vi "Get Transceivers Directory.vi"(8 "error in (no error)":errorcluster, 11 "Transceiver Loader in":refnum<class "Transceiver Loader.lvclass">) -> (0 "error out":errorcluster, 2 "transceivers directory":path, 3 "Transceiver Loader out":refnum<class "Transceiver Loader.lvclass">)   [LabVIEW 2017, in "Data Sharing Framework Core.lvlib" / "Data Sharing Framework Engine.lvlib" / "Transceiver Loader.lvclass"]
uses:
  Transceiver Loader.lvclass
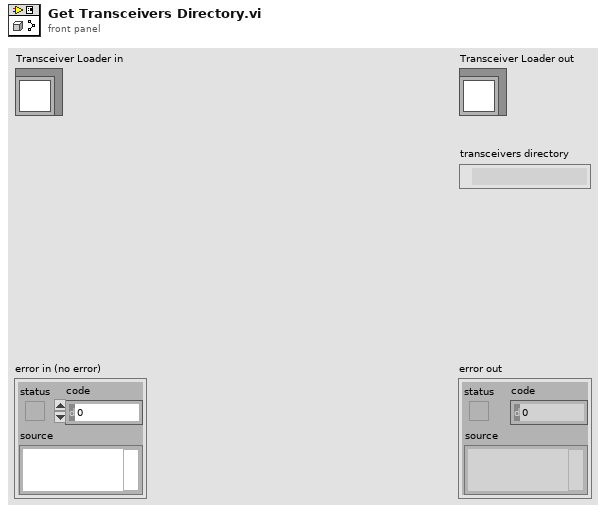
[diagram p1: front panel]
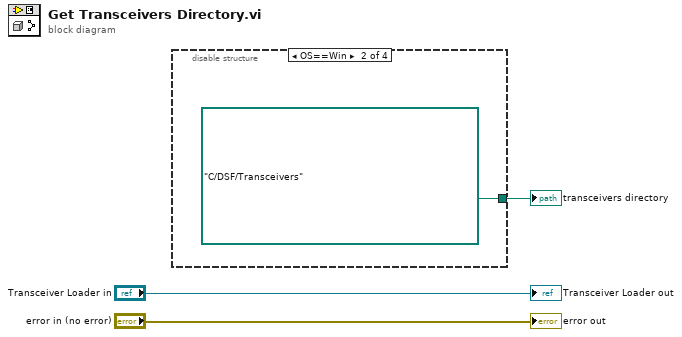
[diagram p0: block diagram]
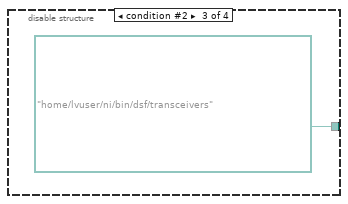
[diagram p3: hidden frame]
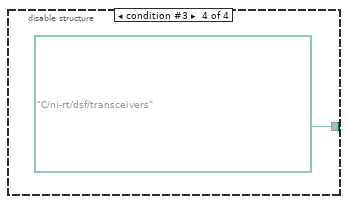
[diagram p4: hidden frame]
diagram:
  n1 = disable-structure shown="OS==Win" {
    disable-tunnel: [_ path "C:/DSF/Transceivers" ("transceivers directory") path "/home/lvuser/ni/bin/dsf/transceivers" ("transceivers directory") path "C:/ni-rt/dsf/transceivers" ("transceivers directory")] -> w1
    frame condition #0 {
    }
    frame condition #1 (active) {
    }
    frame condition #2 {
    }
    frame condition #3 {
    }
  }
  "transceivers directory" <- w1
  "error out" <- "error in (no error)"
  "Transceiver Loader out" <- "Transceiver Loader in"
